vi "Base de datos tirantes.vi"(10 "Tirante":i32, 11 "Semi-Arpa":i32) -> (3 "output cluster":T1)   [LabVIEW 2012]
uses:
  <vilib>/Utility/file.llb/Read From Spreadsheet File (string).vi
  <userlib>/_OpenG.lib/array/array.llb/Search 1D Array (String)__ogtk.vi
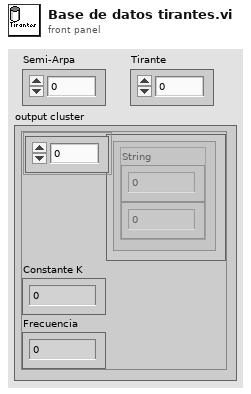
[diagram p1: front panel]
types:
  T1 = cluster{"Array":cluster{"String":dbl, "Numeric Control":u32}[], "Constante K":dbl, "Frecuencia":dbl}
  T2 = cluster{cluster{"String":dbl, u32}[], "Constante K":dbl, "Frecuencia":dbl}
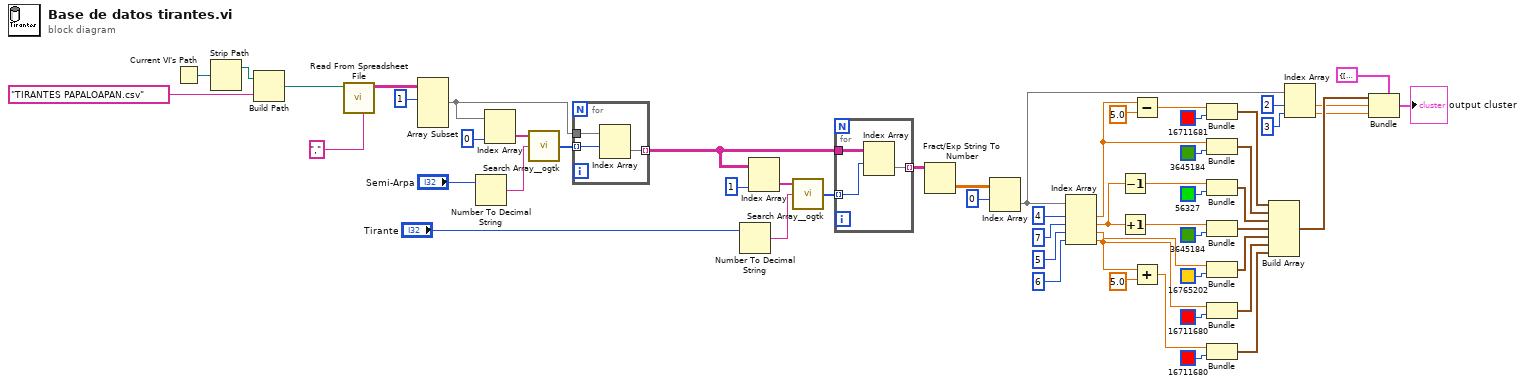
[diagram p0: block diagram]
diagram:
  n1 = Current VI's Path() -> (path=w58:path)
  n2 = Strip Path(path=w58) -> (stripped path=w57:path)  [unwired: 1 out]
  n3 = Build Path(base path=w57, name or relative path="TIRANTES PAPALOAPAN.csv") -> (appended path=w55:path)
  n4 = call-poly <vilib>:"Read From Spreadsheet File.vi"("delimiter (\\t)"="," ("delimiter (\\t)"), "file path (dialog if empty)"=w55) -> ("all rows"=w53:string[][])  [unwired: 5 in, 4 out]
  n5 = Array Subset(array=w53, index (row)=1 ("index")) -> (w45:string[][])  [unwired: 3 in]
  n6 = Number To Decimal String(number="Semi-Arpa") -> (decimal integer string=w47:string)  [unwired: 1 in]
  n7 = Index Array(array=w45, index (col)=0 ("disabled index (col)")) -> (element=w48:string[])  [unwired: 1 in]
  n8 = call-poly <userlib>:"Search Array__ogtk.vi"("Array"=w48, "Element Data"=w47) -> ("Indices of Elements"=w46:i32[])  [unwired: 7 in]
  n9 = for {
    tunnel: w46 -> [w60] mode=indexing
    tunnel: w45 -> [w61]
    tunnel: [w59] -> w41 mode=indexing
    n10 = Index Array(array=w61, index (row)=w60) -> (element=w59:string[])  [unwired: 1 in]
  }
  n11 = Number To Decimal String(number="Tirante") -> (decimal integer string=w42:string)  [unwired: 1 in]
  n12 = Index Array(array=w41, index (col)=1 ("disabled index (col)")) -> (element=w43:string[])  [unwired: 1 in]
  n13 = call-poly <userlib>:"Search Array__ogtk.vi"("Array"=w43, "Element Data"=w42) -> ("Indices of Elements"=w40:i32[])  [unwired: 7 in]
  n14 = for {
    tunnel: w40 -> [w63] mode=indexing
    tunnel: w41 -> [w64]
    tunnel: [w62] -> w39 mode=indexing
    n15 = Index Array(array=w64, index (row)=w63) -> (element=w62:string[])  [unwired: 1 in]
  }
  n16 = Fract/Exp String To Number(string=w39) -> (number=w38:dbl[][])  [unwired: 3 in, 1 out]
  n17 = Index Array(array=w38, index (row)=0) -> (element=w8:dbl[])  [unwired: 1 in]
  n18 = Index Array(array=w8, index #1=4 ("index"), index #2=7 ("index"), index #3=5 ("index"), index #4=6 ("index")) -> (element #1=w31:dbl, element #2=w24:dbl, element #3=w19:dbl, element #4=w14:dbl)
  n19 = Decrement(x=w24) -> (x-1=w27:dbl)
  n20 = Increment(x=w24) -> (x+1=w23:dbl)
  n21 = Subtract(x=w31, y=5.0) -> (x-y=w33:dbl)
  n22 = Add(x=w14, y=5.0) -> (x+y=w11:dbl)
  n23 = Bundle(w33, u32 16711681) -> (w32:cluster{dbl, u32})  [unwired: 1 in]
  n24 = Bundle("String"=w31, u32 3645184) -> (w29:cluster{"String":dbl, u32})  [unwired: 1 in]
  n25 = Bundle(w27, u32 56327) -> (w25:cluster{dbl, u32})  [unwired: 1 in]
  n26 = Bundle(w23, u32 3645184) -> (w21:cluster{dbl, u32})  [unwired: 1 in]
  n27 = Bundle("String"=w19, u32 16765202) -> (w17:cluster{"String":dbl, u32})  [unwired: 1 in]
  n28 = Bundle("String"=w14, u32 16711680) -> (w12:cluster{"String":dbl, u32})  [unwired: 1 in]
  n29 = Bundle(w11, u32 16711680) -> (w9:cluster{dbl, u32})  [unwired: 1 in]
  n30 = Build Array(w32, w29, w25, w21, w17, w12, w9) -> (w5:cluster{"String":dbl, u32}[])
  n31 = Index Array(array=w8, index #1=2 ("index"), index #2=3 ("index")) -> (element #1=w4:dbl, element #2=w3:dbl)
  n32 = Bundle(cluster=T2 {[], "Constante K"=0.0, "Frecuencia"=0.0}, w5, "Constante K"=w4, "Frecuencia"=w3) -> (→"output cluster":T2)
